vi "Hardware Device Subpanel.vi"(1 "Data Types":T2(array[cluster]), 2 "Data Names&Defaults":string[][](array[string])) -> (0 "Data Names&Data":string[][](array[string]))   [LabVIEW 2016, in "TSPopup.lvlib"]
doc: "Demo showing dynamically changing data types and working with a tree.\n\nType Sensitive Popup \nCopyright © 2007, J. David Saunders\nAll rights reserved."
uses:
  <userlib>/TSPopup/TSPopup.lvlib
  <userlib>/TSPopup/TSPopup.Popup Cluster.ctl
  <userlib>/TSPopup/TSPopup.lvclass
  <userlib>/TSPopup/TSPopup.Grid.Cell Info.ctl
  <userlib>/TSPopup/TSPopup.Data Type.ctl
panel:
  in  "Popups":T1 {"Boolean" items=["False", "True"]}
  in  "Cancel Button":bool
  in  "OK Button":bool
  in  "Data List":i32(listbox)
  # "Type Sensitive Popup \nCopyright © 2007, J. David Saunders\nAll rights reserved."
  # "Type Sensitive\nPopup"
  # "Boolean Colors"
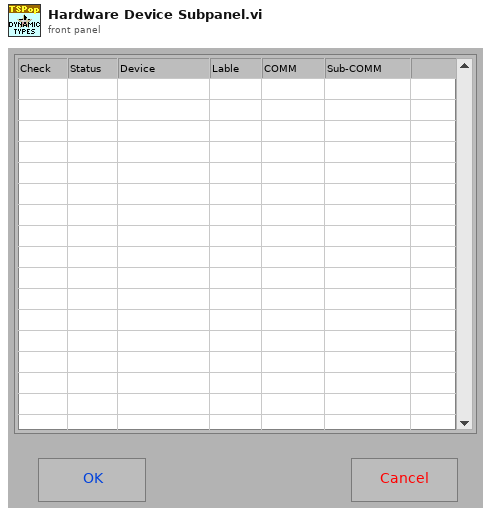
[diagram p1: front panel]
types:
  T1 = typedef "TSPopup.lvlib/TSPopup.lvclass/TSPopup.Popup Cluster.ctl" = cluster{"Unknown":bool, "Unknown 2":bool, "String":string, "Integer":i32, "Float":dbl, "Color":u32, "Boolean":u32, "Ring":u32, "Captioned String":cluster{"String":string, "OK":bool, "Cancel":bool}, "Captioned Integer":cluster{"First":i32, "OK":bool, "Cancel":bool}, "Boolean Colors":cluster{"False":cluster{"FG":u32, "BG":u32}, "True":cluster{"FG":u32, "BG":u32}, "T  to  F":cluster{"FG":u32, "BG":u32}, "F  to  T":cluster{"FG":u32, "BG":u32}, "OK":bool, "Cancel":bool}, "2-Int Cluster":cluster{"First":i32, "Second":i32, "OK":bool, "Cancel":bool}, "4-Int Cluster":cluster{"First":i32, "Second":i32, "Third":i32, "Fourth":i32, "OK":bool, "Cancel":bool}, "check":bool}
  T2 = cluster{"Data Type":string, "Caption/Ring Strings":string[]}[]
  T3 = typedef "TSPopup.lvlib/TSPopup.lvclass/TSPopup.Grid.Cell Info.ctl" = cluster{"Tag":string, "Row":i32, "Column":i32, "In Symbol?":bool, "In Data?":bool, "Cell String":string, "Ctl Refnum":refnum<vi>, "Prop Type":T4, "Ring Strings":string[]}
  T4 = typedef "TSPopup.lvlib/TSPopup.lvclass/TSPopup.Data Type.ctl" = enum16{"Unkown", "NO POPUP", "String", "Integer", "Float", "Color", "Boolean", "Ring", "Captioned String", "Captioned Integer", "Button Color", "2 Int Cluster", "4 Int Cluster", "check"}
  T5 = typedef "LVPoint32TypeDef.ctl" = cluster{"Horizontal":i32, "Vertical":i32}
  T6 = typedef "TSPopup.lvlib/TSPopup.lvclass/TSPopup.Popup Call Parameters.ctl" = cluster{"Prop Type":T4, "Initial Value":variant, "Caption Strings":string[], "Ring Strings":string[], "Cell Rect":cluster{"left":i16, "top":i16, "right":i16, "bottom":i16}, "Mouse Coords":cluster{"x":i16, "y":i16}, "Call Data":variant}
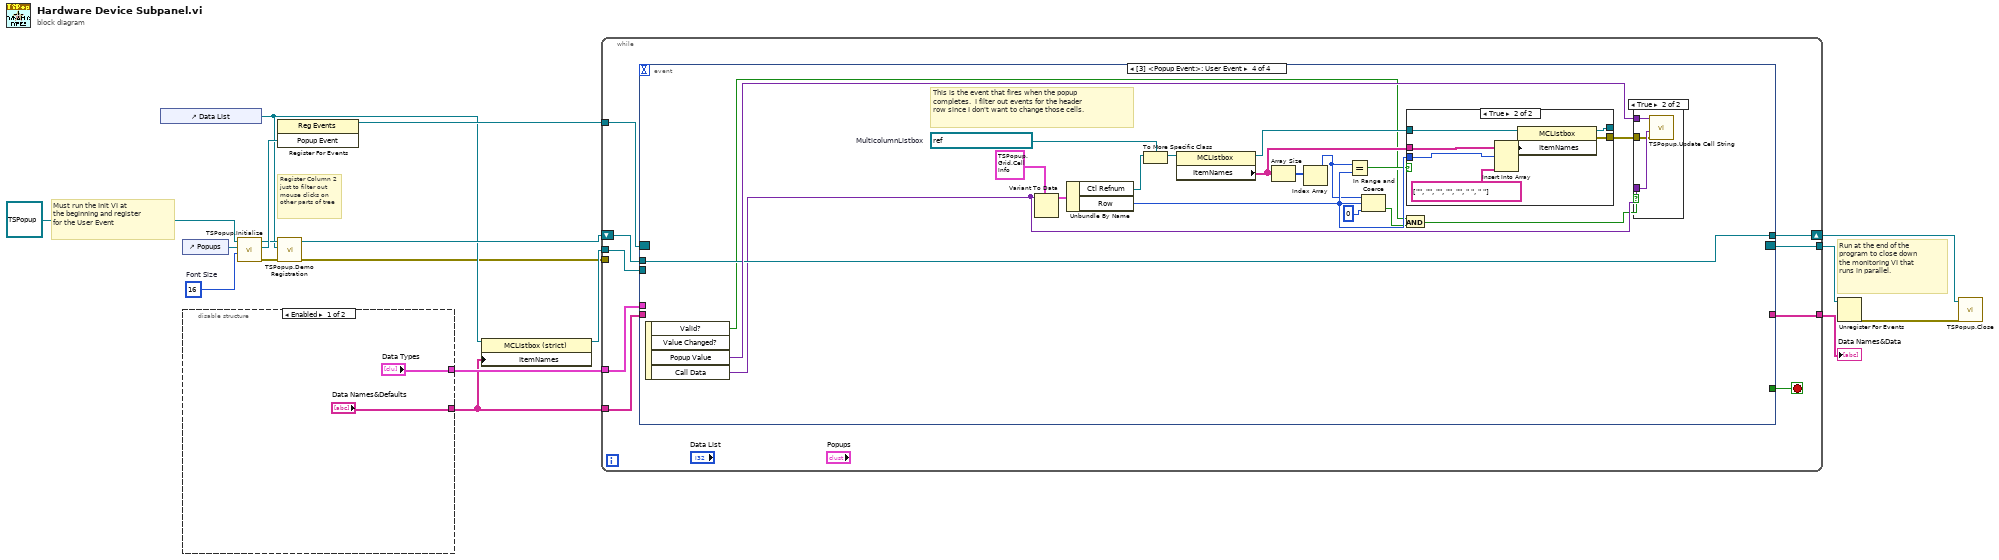
[diagram p0: block diagram]
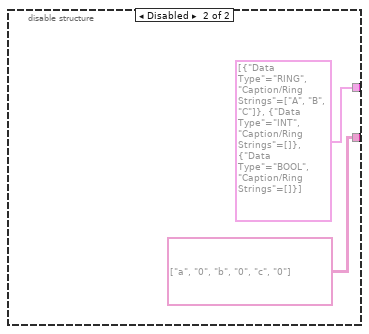
[diagram p2: hidden frame]
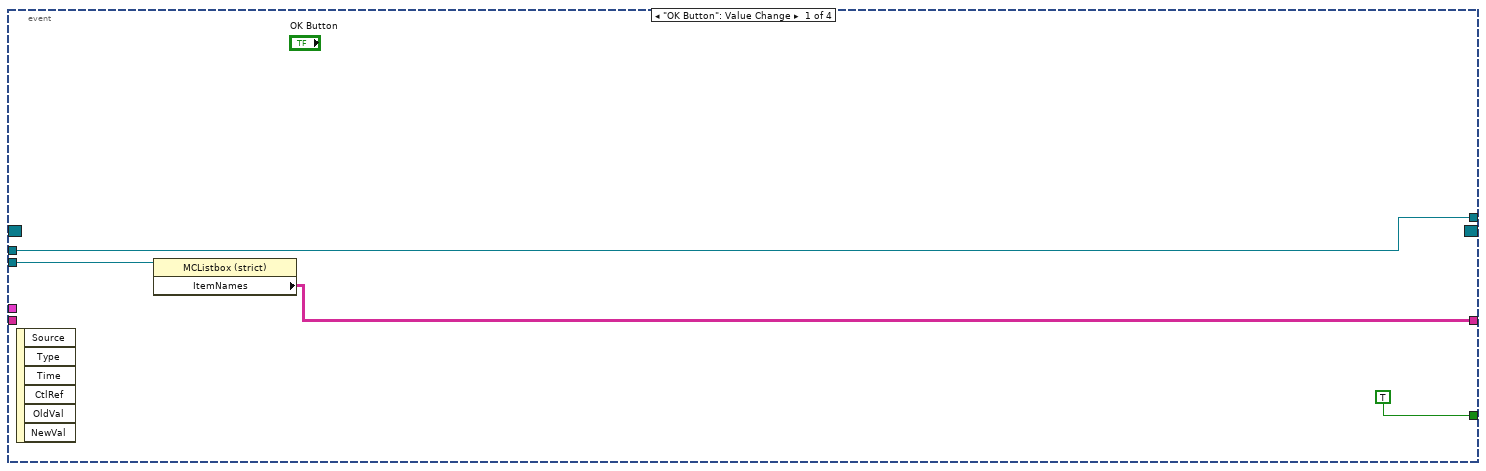
[diagram p3: hidden frame]
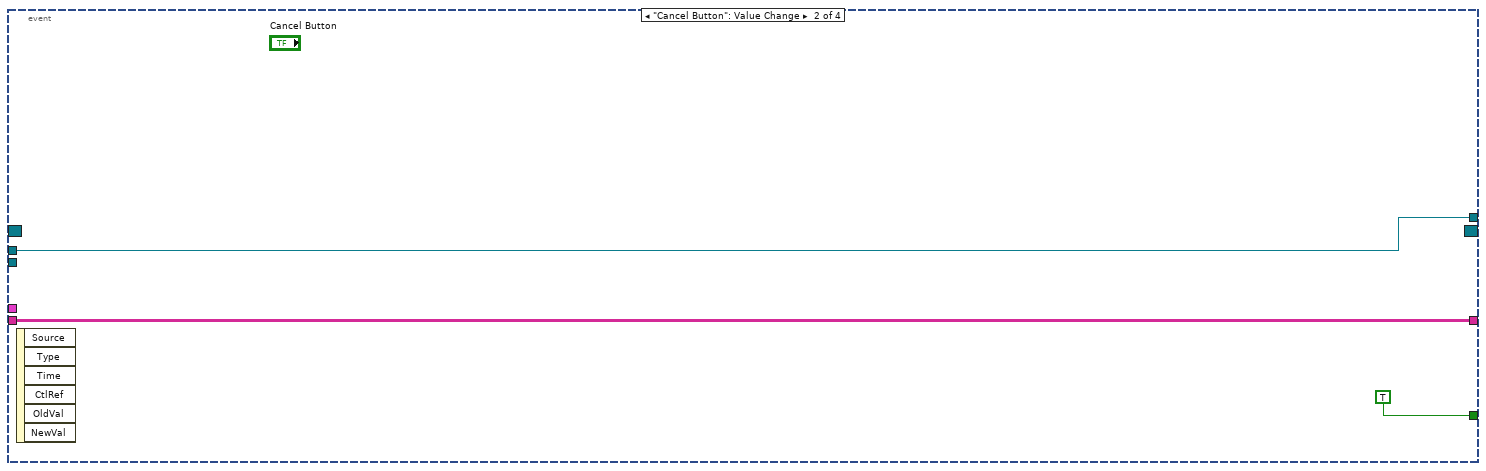
[diagram p4: hidden frame]
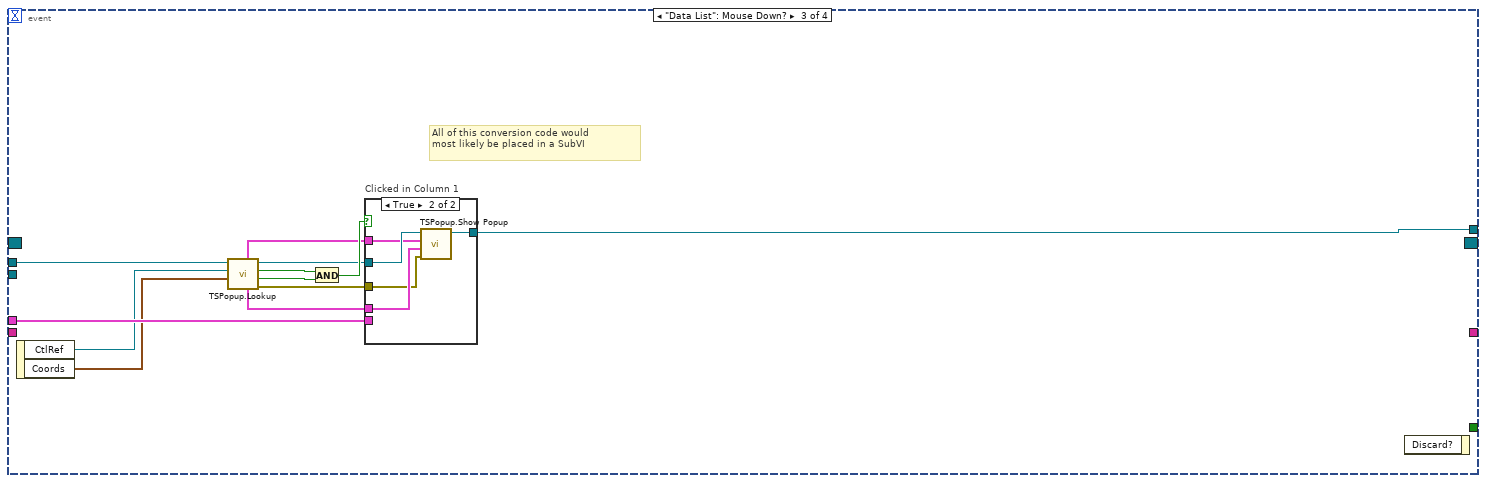
[diagram p5: hidden frame]
diagram:
  w12 = u32 16  # Font Size
  # "Register Column 2\njust to filter out\nmouse clicks on\nother parts of tree"
  # "Run at the end of the\nprogram to close down\nthe monitoring VI that\nruns in parallel."
  # "Must run the Init VI at\nthe beginning and register\nfor the User Event"
  n1 = control-ref of="Data List"() -> (w3:refnum<vi>)
  n2 = control-ref of="Popups"() -> (w9:refnum<vi>)
  n3 = disable-structure shown="Enabled" {
    disable-tunnel: ["Data Types" T2 [{"Data Type"="RING", "Caption/Ring Strings"=["A", "B", "C"]}, {"Data Type"="INT", "Caption/Ring Strings"=[]}, {"Data Type"="BOOL", "Caption/Ring Strings"=[]}] ("Data Types")] -> w14
    disable-tunnel: ["Data Names&Defaults" string[][] [["a", "0"], ["b", "0"], ["c", "0"]] ("Data Names&Defaults")] -> w6
    frame Enabled {
    }
    frame Disabled {
    }
  }
  n4 = call <userlib>:"TSPopup.Initialize.vi"("Font Size"=w12, "Popup Cluster Ref"=w9, "TSPopup in"=refnum<class "TSPopup.lvclass"> refnum ("TSPopup.lvclass")) -> ("error out"=w2:errorcluster, "Popup Event"=w11:refnum<user-event>, "TSPopup out"=w5:refnum<class "TSPopup.lvclass">)  [unwired: 6 in]
  n5 = register-events(w11) -> (reference out=w17:refnum<event-registration>)  [unwired: 2 in, 1 out]
  n6 = call <userlib>:"TSPopup.Demo Registration.vi"("TSPopup in"=w5, "Signal Settings ref"=w3, "error in (no error)"=w2) -> ("TSPopup out"=w4:refnum<class "TSPopup.lvclass">, "error out"=w1:errorcluster)  [unwired: 6 in]
  n7 = property class="MCListbox (strict)"(reference=w3, "ItemNames"=w6) -> (reference out=w8:refnum<vi>)  [unwired: 1 in, 1 out]
  n8 = while {
    tunnel: w17 -> [w30]
    tunnel: [w29] -> w16
    tunnel: w14 -> [w27]
    tunnel: w1 -> [_]
    shift-right: [w25] -> w10
    shift-left: w4 -> [w26]
    tunnel: w8 -> [w24]
    tunnel: [w23] -> w7
    tunnel: w6 -> [w22]
    stop <- w28 stop-if-true
    n9 = event shown="[3] <Popup Event>: User Event" {
      selector: w30 -> [_ _ _ _]
      dyn-events: [_ _ _ _] -> w29
      timeout: _ -> [_ _ _ _]
      tunnel: [TRUE TRUE _ _] -> w28
      tunnel: w27 -> [_ _ w48 _]
      tunnel: w26 -> [w33 w36 w40 w73]
      tunnel: [w33 w36 w38 w73] -> w25
      tunnel: w24 -> [w32 _ _ _]
      tunnel: [w31 w35 _ _] -> w23
      tunnel: w22 -> [_ w35 _ _]
      event "OK Button": Value Change {
        n10 = event-data() -> ()  [unwired: 1 in, 6 out]
        n11 = property class="MCListbox (strict)"(reference=w32) -> ("ItemNames"=w31:string[][])  [unwired: 1 in, 2 out]
      }
      event "Cancel Button": Value Change {
        n12 = event-data() -> ()  [unwired: 1 in, 6 out]
      }
      event "Data List": Mouse Down? {
        # "All of this conversion code would\nmost likely be placed in a SubVI"
        n13 = event-data() -> ("CtlRef"=w47:refnum<vi>, "Coords"=w46:T5)  [unwired: 1 in]
        n14 = call <userlib>:"TSPopup.Lookup.vi"("Point"=w46, "Ctl Refnum"=w47, "TSPopup in"=w40) -> ("error out"=w42:errorcluster, "In Bounds?"=w43:bool, "Found"=w44:bool, "TSPopup out"=w39:refnum<class "TSPopup.lvclass">, "Cell Info (Call data)"=w41:T3, "Popup Parameters"=w45:T6)  [unwired: 3 in]
        n15 = And(x=w44, y=w43) -> (x .and. y?=w49:bool)
        n16 = case "Clicked in Column 1" shown="True" w49 {
          tunnel: w45 -> [_ w51]
          tunnel: w41 -> [_ w53]
          tunnel: w42 -> [_ w52]
          tunnel: w48 -> [_ _]
          tunnel: w39 -> [w50 w55]
          tunnel: [w50 w54] -> w38
          frame False {
          }
          frame True {
            n17 = call <userlib>:"TSPopup.Show Popup.vi"("error in (no error)"=w52, "Call Data (ignore if empty)"=w53, "Popup Parameters"=w51, "TSPopup in"=w55) -> ("TSPopup out"=w54:refnum<class "TSPopup.lvclass">)  [unwired: 6 in, 1 out]
          }
        }
        n18 = event-data() -> ()  [unwired: 2 in, 1 out]
      }
      event User Event {
        w68 = refnum<vi> refnum  # MulticolumnListbox
        # "This is the event that fires when the popup\ncompletes.  I filter out events for the header\nrow since I don't want to change those cells."
        n19 = event-data() -> ("Valid?"=w58:bool, "Popup Value"=w74:variant, "Call Data"=w59:variant)  [unwired: 1 in, 1 out]
        n20 = Variant To Data(type=T3 {"Tag"="", "Row"=0, "Column"=0, "In Symbol?"=FALSE, "In Data?"=FALSE, "Cell String"="", "Ctl Refnum"=refnum, "Prop Type"=enum."Unkown", "Ring Strings"=[]} ("Cell Info (type only)"), Variant=w59) -> (data=w72:T3)  [unwired: 1 in, 1 out]
        n21 = Unbundle By Name(w72) -> ("Ctl Refnum"=w70:refnum<vi>, "Row"=w63:i32)
        n22 = To More Specific Class(target class=w68, reference=w70) -> (specific class reference=w69:refnum<vi>)  [unwired: 1 in, 1 out]
        n23 = property class="MCListbox"(reference=w69) -> (reference out=w65:refnum<vi>, "ItemNames"=w66:string[][])  [unwired: 1 in, 1 out]
        n24 = Array Size(array=w66) -> (size(s)=w67:i32[])
        n25 = Index Array(array=w67) -> (element=w62:i32)  [unwired: 1 in]
        n26 = Equal?(x=w62, y=w63) -> (x = y?=w60:bool)
        n27 = In Range and Coerce(upper limit=w62, x=w63, lower limit=0) -> (In Range?=w61:bool)  [unwired: 1 out]
        n28 = And(x=w58, y=w61) -> (x .and. y?=w57:bool)
        n29 = case shown="True" w60 {
          tunnel: w66 -> [_ w82]
          tunnel: w63 -> [_ w81]
          tunnel: w65 -> [w75 w79]
          tunnel: [_ w77] -> w56
          tunnel: [w75 w76] -> _
          frame False {
          }
          frame True {
            n30 = Insert Into Array(array=w82, index (row)=w81, new element=string[] ["", "", "", "", "", " ", " "] ("new element/subarray")) -> (w78:string[][])  [unwired: 1 in]
            n31 = property class="MCListbox"(reference=w79, "ItemNames"=w78) -> (reference out=w76:refnum<vi>, error out=w77:errorcluster)  [unwired: 1 in]
          }
        }
        n32 = case shown="True" w57 {
          tunnel: w74 -> [_ w84]
          tunnel: w59 -> [_ w85]
          tunnel: w56 -> [_ w83]
          frame False {
          }
          frame True {
            n33 = call <userlib>:"TSPopup.Update Cell String.vi"("error in (no error)"=w83, "Call Data (must be Cell Info cluster)"=w85, "Popup Value"=w84) -> ()  [unwired: 8 in, 1 out]
          }
        }
      }
    }
  }
  "Data Names&Data" <- w7
  n34 = Unregister For Events(event registration refnum=w16) -> (error out=w15:errorcluster)  [unwired: 1 in]
  n35 = call <userlib>:"TSPopup.Close.vi"("error in (no error)"=w15, "TSPopup in"=w10) -> ()  [unwired: 8 in, 2 out]
